vi "OEE_SCREEN_2_recolor.vi"(7 "SCREEN_2_recolor_references":T2, 8 "error_in":errorcluster, 11 "SCREEN_2":T1={"header_part_no"="-", "header_customer"="-", "performance_percentage"="-", "performance_target"="-", "performance_actual"="-", "performance_header"="PERFORMANCE", "performance_header_target"="TARGET", "performance_header_actual"="ACTUAL"}) -> (0 "error_out":errorcluster)   [LabVIEW 2019]
uses:
  typedef/SCREEN_2_recolor_references.ctl
  typedef/SCREEN_2.ctl
panel:
  # "Performance Data Output Board #2"
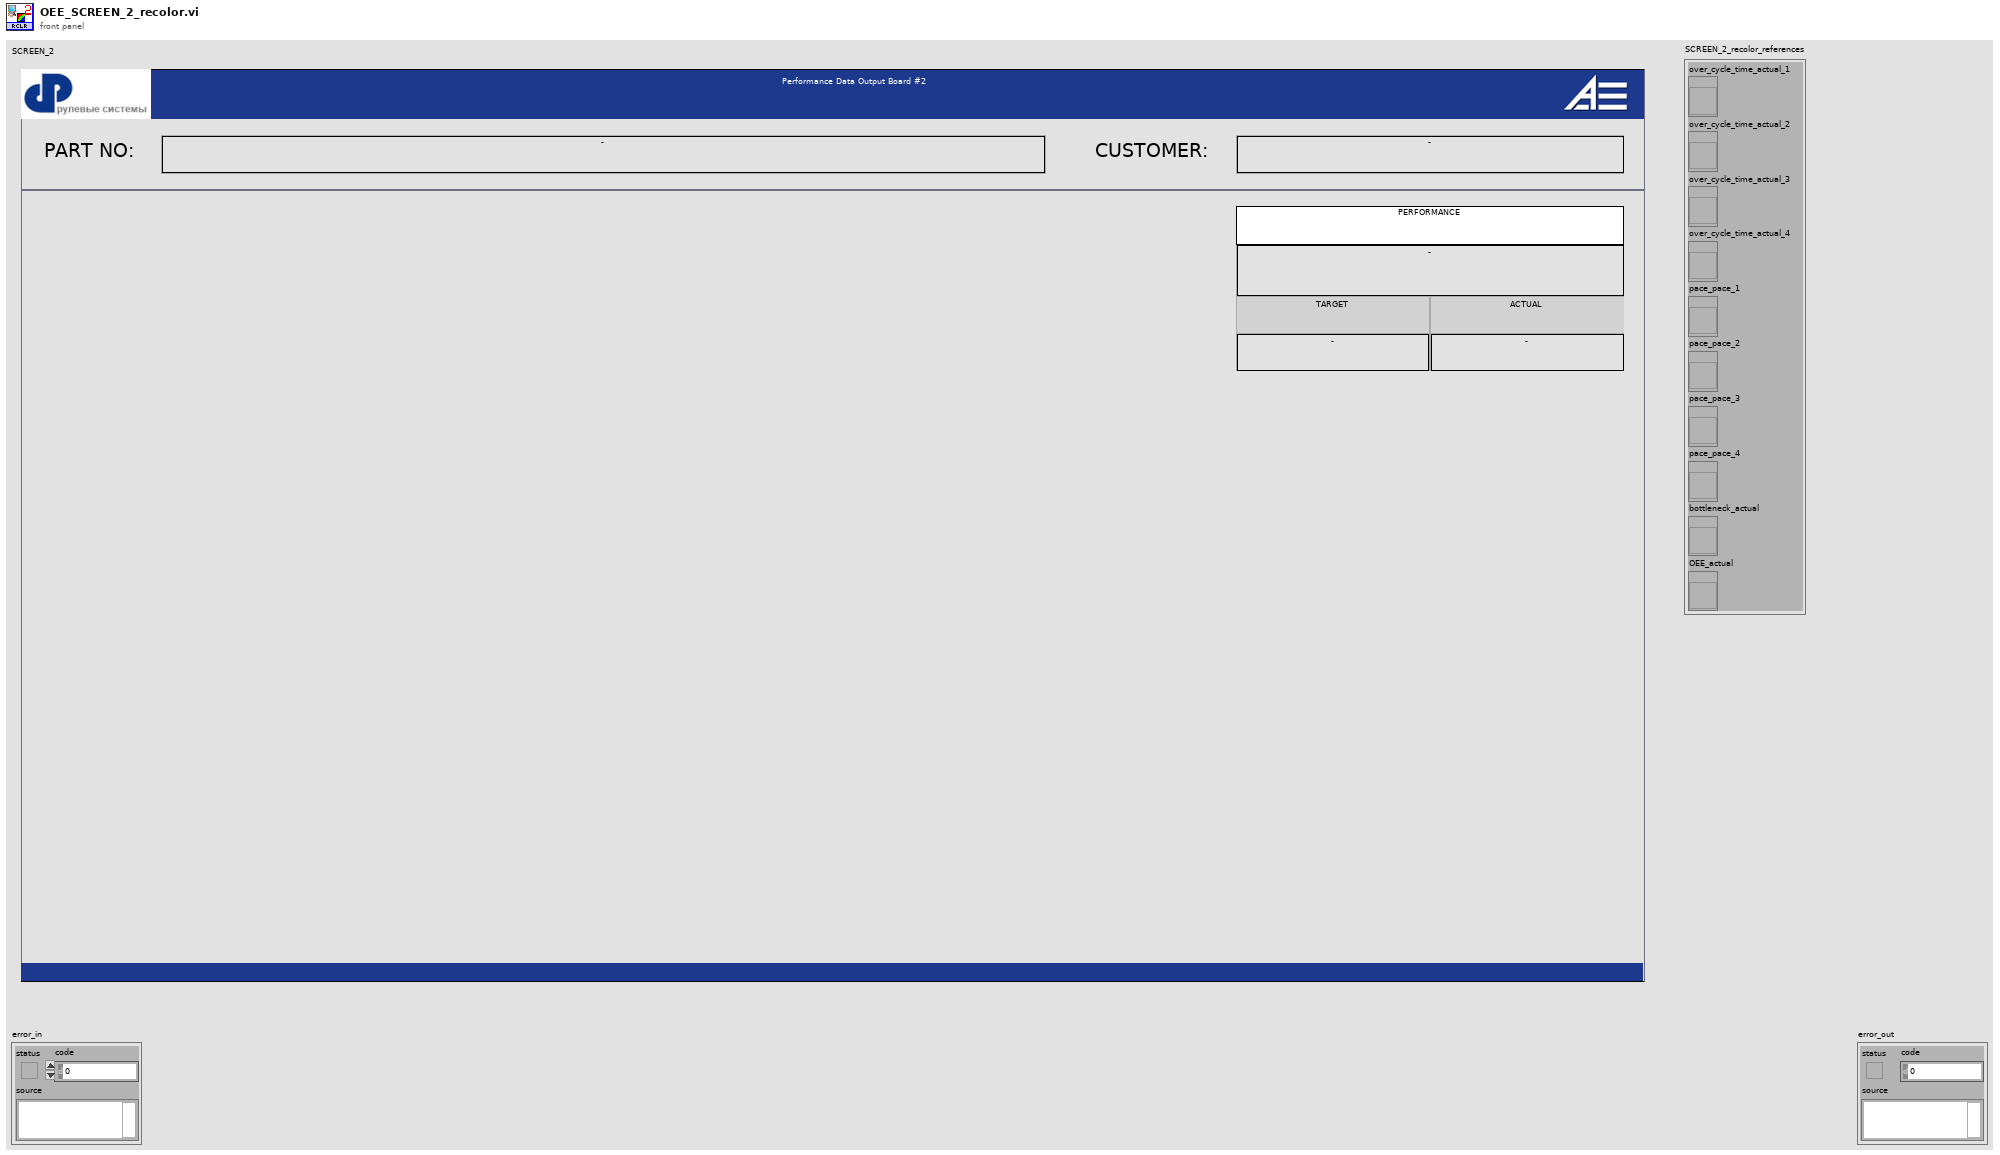
[diagram p1: front panel]
types:
  T1 = typedef "SCREEN_2.ctl" = cluster{"header_part_no":string, "header_customer":string, "performance_percentage":string, "performance_target":string, "performance_actual":string, "performance_header":string, "performance_header_target":string, "performance_header_actual":string}
  T2 = typedef "SCREEN_2_recolor_references.ctl" = cluster{"over_cycle_time_actual_1":refnum<vi>, "over_cycle_time_actual_2":refnum<vi>, "over_cycle_time_actual_3":refnum<vi>, "over_cycle_time_actual_4":refnum<vi>, "pace_pace_1":refnum<vi>, "pace_pace_2":refnum<vi>, "pace_pace_3":refnum<vi>, "pace_pace_4":refnum<vi>, "bottleneck_actual":refnum<vi>, "OEE_actual":refnum<vi>}
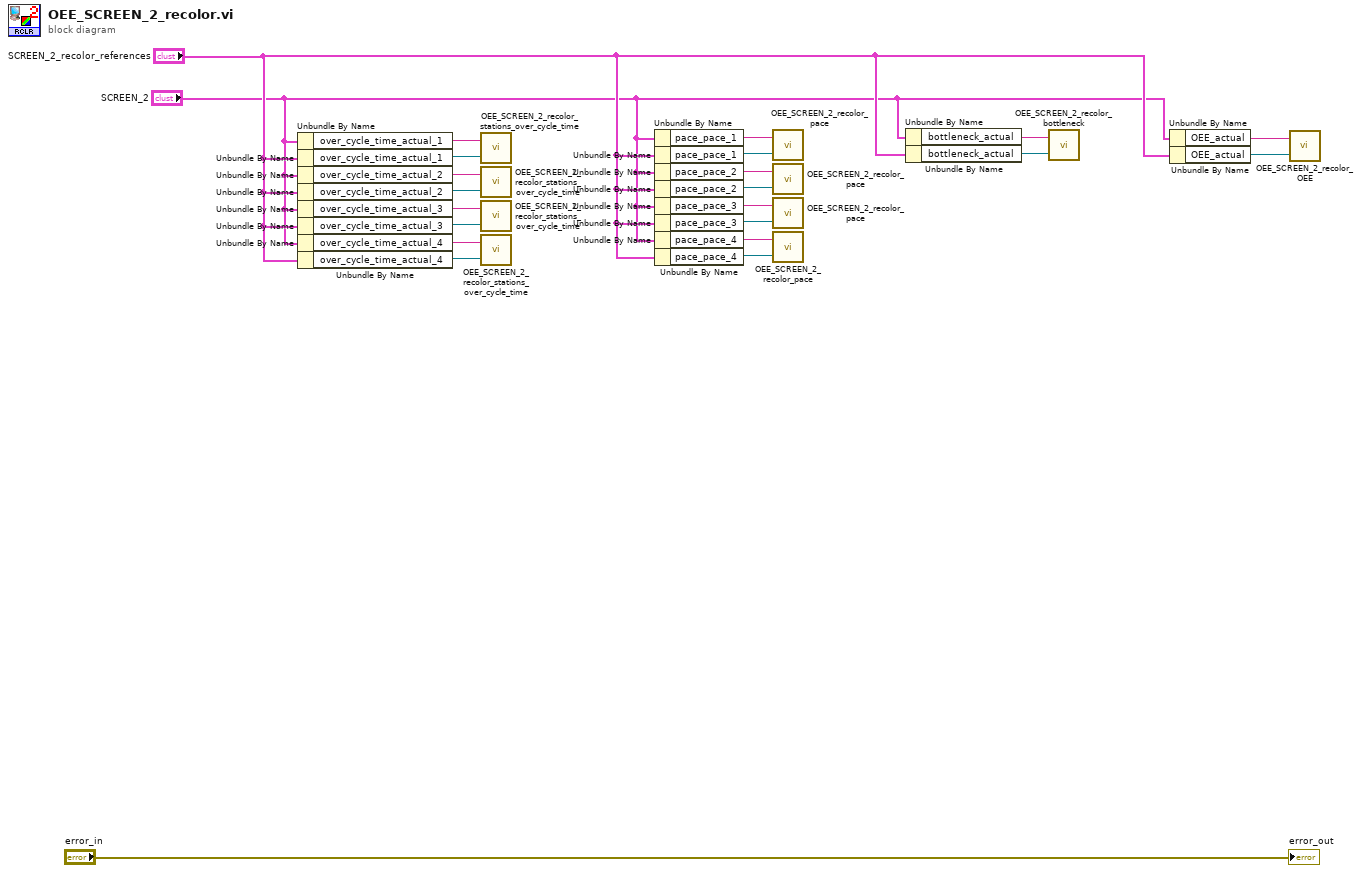
[diagram p0: block diagram]
diagram:
  n1 = Unbundle By Name("SCREEN_2") -> ("over_cycle_time_actual_1"=w20:string)
  n2 = Unbundle By Name("SCREEN_2_recolor_references") -> ("over_cycle_time_actual_1"=w19:refnum<vi>)
  n3 = Unbundle By Name("SCREEN_2") -> ("over_cycle_time_actual_2"=w18:string)
  n4 = Unbundle By Name("SCREEN_2_recolor_references") -> ("over_cycle_time_actual_2"=w17:refnum<vi>)
  n5 = Unbundle By Name("SCREEN_2") -> ("over_cycle_time_actual_3"=w16:string)
  n6 = Unbundle By Name("SCREEN_2_recolor_references") -> ("over_cycle_time_actual_3"=w15:refnum<vi>)
  n7 = Unbundle By Name("SCREEN_2") -> ("over_cycle_time_actual_4"=w14:string)
  n8 = Unbundle By Name("SCREEN_2_recolor_references") -> ("over_cycle_time_actual_4"=w13:refnum<vi>)
  n9 = call "OEE_SCREEN_2_recolor_stations_over_cycle_time.vi"("over_cycle_time_actual_field_reference"=w19, "over_cycle_time_actual"=w20) -> ()  [unwired: 1 in]
  n10 = call "OEE_SCREEN_2_recolor_stations_over_cycle_time.vi"("over_cycle_time_actual_field_reference"=w17, "over_cycle_time_actual"=w18) -> ()  [unwired: 1 in]
  n11 = call "OEE_SCREEN_2_recolor_stations_over_cycle_time.vi"("over_cycle_time_actual_field_reference"=w15, "over_cycle_time_actual"=w16) -> ()  [unwired: 1 in]
  n12 = call "OEE_SCREEN_2_recolor_stations_over_cycle_time.vi"("over_cycle_time_actual_field_reference"=w13, "over_cycle_time_actual"=w14) -> ()  [unwired: 1 in]
  n13 = Unbundle By Name("SCREEN_2") -> ("pace_pace_1"=w12:string)
  n14 = Unbundle By Name("SCREEN_2_recolor_references") -> ("pace_pace_1"=w11:refnum<vi>)
  n15 = Unbundle By Name("SCREEN_2") -> ("pace_pace_2"=w10:string)
  n16 = Unbundle By Name("SCREEN_2_recolor_references") -> ("pace_pace_2"=w9:refnum<vi>)
  n17 = Unbundle By Name("SCREEN_2") -> ("pace_pace_3"=w8:string)
  n18 = Unbundle By Name("SCREEN_2_recolor_references") -> ("pace_pace_3"=w7:refnum<vi>)
  n19 = Unbundle By Name("SCREEN_2") -> ("pace_pace_4"=w6:string)
  n20 = Unbundle By Name("SCREEN_2_recolor_references") -> ("pace_pace_4"=w5:refnum<vi>)
  n21 = call "OEE_SCREEN_2_recolor_pace.vi"("pace_field_reference"=w11, "pace_value"=w12) -> ()  [unwired: 1 in]
  n22 = call "OEE_SCREEN_2_recolor_pace.vi"("pace_field_reference"=w9, "pace_value"=w10) -> ()  [unwired: 1 in]
  n23 = call "OEE_SCREEN_2_recolor_pace.vi"("pace_field_reference"=w7, "pace_value"=w8) -> ()  [unwired: 1 in]
  n24 = call "OEE_SCREEN_2_recolor_pace.vi"("pace_field_reference"=w5, "pace_value"=w6) -> ()  [unwired: 1 in]
  n25 = Unbundle By Name("SCREEN_2") -> ("bottleneck_actual"=w4:string)
  n26 = Unbundle By Name("SCREEN_2_recolor_references") -> ("bottleneck_actual"=w3:refnum<vi>)
  n27 = call "OEE_SCREEN_2_recolor_bottleneck.vi"("bottleneck_field_reference"=w3, "bottleneck_value"=w4) -> ()  [unwired: 1 in]
  n28 = Unbundle By Name("SCREEN_2") -> ("OEE_actual"=w2:string)
  n29 = Unbundle By Name("SCREEN_2_recolor_references") -> ("OEE_actual"=w1:refnum<vi>)
  n30 = call "OEE_SCREEN_2_recolor_OEE.vi"("OEE_actual_field_reference"=w1, "OEE_actual_value"=w2) -> ()  [unwired: 1 in]
  "error_out" <- "error_in"
